vi "read big txt - rev1_from folder.vi"(11 "파일 경로(대화 상자 사용)":path) -> (3 "배열":string[](array[string]))   [LabVIEW 2015]
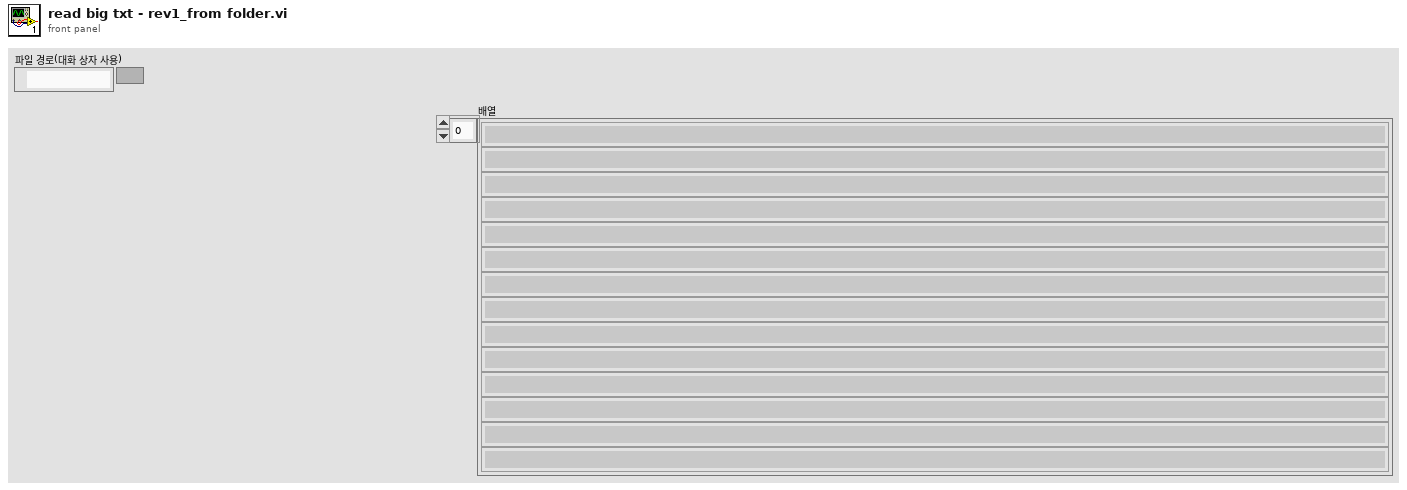
[diagram p1: front panel]
types:
  T1 = enum16{"open", "replace", "create", "open or create", "replace or create", "replace or create with confirmation"}
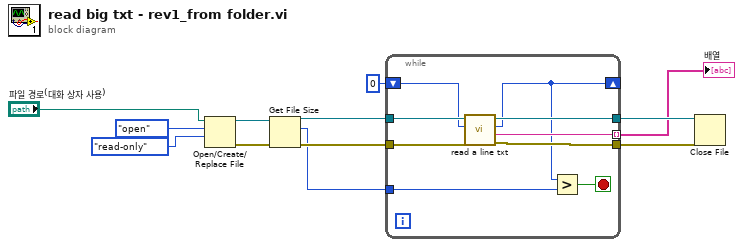
[diagram p0: block diagram]
diagram:
  n1 = Open/Create/Replace File(file path (use dialog)="파일 경로(대화 상자 사용)", operation (0:open)=T1."open" ("동작(0:open)"), access (0:read/write)=enum16{"read/write", "read-only", "write-only"}."read-only" ("접근(0:읽기/쓰기)")) -> (refnum out=w10:refnum<file>, error out=w9:errorcluster)  [unwired: 3 in, 1 out]
  n2 = Get File Size(file=w10, error in=w9) -> (refnum out=w8:refnum<file>, size (in bytes)=w2:i64, 0:w7:errorcluster)
  n3 = while {
    tunnel: [w21] -> w3 mode=indexing
    tunnel: w8 -> [w20]
    tunnel: w7 -> [w19]
    tunnel: [w18] -> w5
    tunnel: [w17] -> w4
    shift-right: [w15] -> _
    shift-left: i64 0 ("last offset+1") -> [w16]
    tunnel: w2 -> [w13]
    stop <- w14 stop-if-true
    n4 = call "read a line txt.vi"("에러 입력"=w19, "오프셋(바이트) (0)"=w16, "참조 번호"=w20) -> ("error out"=w17:errorcluster, "문자열"=w21:string, "last offset"=w15:i64, "refnum out"=w18:refnum<file>)  [unwired: 5 in]
    n5 = Greater?(x=w15, y=w13) -> (0:w14:bool)
  }
  "배열" <- w3
  n6 = Close File(refnum=w5, error in=w4) -> ()  [unwired: 2 out]
